vi "offsetArrayIndex.vi"(11 "y_offset_host array":fxp<+/-,16,8>[](array[numeric])) -> (3 "index":i32)   [LabVIEW 2020]
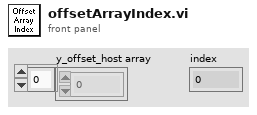
[diagram p1: front panel]
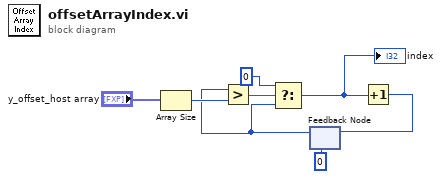
[diagram p0: block diagram]
diagram:
  n1 = Array Size(array="y_offset_host array") -> (size(s)=w5:i32)
  n2 = feedback #1(0 ("x")) -> (w1:i32)
  n3 = Greater?(x=w1, y=w5) -> (0:w6:bool)
  n4 = Select(t=0, s=w6, f=w1) -> (s? t:f=w3:i32)
  "index" <- w3
  n5 = Increment(x=w3) -> (x+1=w2:i32)
  n6 = feedback-in #1(w2) -> ()
